vi "Calculate Spring Constant.vi"   [LabVIEW 2013]
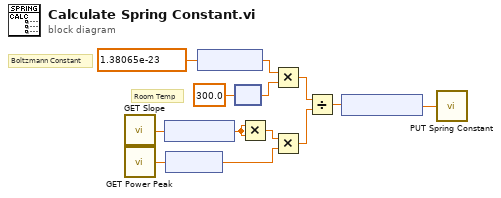
[diagram p0: block diagram]
diagram:
  # "Room Temp"
  # "Boltzmann Constant"
  n1 = call "GET Slope.vi"() -> ("Slope"=w9:dbl)
  n2 = call "GET Power Peak.vi"() -> ("Power Peak"=w8:dbl)
  n3 = node(w9) -> (w3:dbl[unit])
  n4 = node(w8) -> (w7:dbl[unit])
  n5 = node(1.38065e-23) -> (w12:dbl[unit])
  n6 = node(300.0) -> (w13:dbl[unit])
  n7 = Multiply(x=w3, y=w3) -> (x*y=w2:dbl[unit])
  n8 = Multiply(x=w12, y=w13) -> (x*y=w4:dbl[unit])
  n9 = Multiply(x=w2, y=w7) -> (x*y=w6:dbl[unit])
  n10 = Divide(x=w4, y=w6) -> (x/y=w5:dbl[unit])
  n11 = node(w5) -> (w1:dbl)
  n12 = call "PUT Spring Constant.vi"("Spring Constant"=w1) -> ()
